vi "Read DisplayConfig.vi"(8 "error in":errorcluster caption="错误输入（无错误）", 11 "PCM PanelSplit 输入":refnum<class "PCM PanelSplit.lvclass"> caption="DNL_LabVIEW Object in") -> (0 "error out":errorcluster caption="错误输出", 2 "Display Config":T1={"Display Mode"=enum."时域", "ChTag[]"=[], "window"=1, "Range"={"Minimum"=0.0, "Maximum"=0.0, "Increment"=0.0, "Minor Increment"=0.0, "Start"=0.0}} {"window" items=["Rectangle"=0, "Hanning"=1, "Hamming"=2, "Blackman-Harris"=3, "Exact Blackman"=4, "Blackman"=5, "Flat Top"=6, "4 Term B-Harris "=7, "7 Term B-Harris"=8, "Low Sidelobe"=9, "Blackman Nuttall"=11, "Triangle"=30, "Bartlett-Hanning"=31, "Bohman"=32, "Parzen"=33, "Welch"=34, "Kaiser"=60, "Dolph-Chebyshev"=61, "Gaussian"=62]}, 3 "PCM PanelSplit 输出":refnum<class "PCM PanelSplit.lvclass"> caption="DNL_LabVIEW Object out")   [LabVIEW 2016, in "PCM PanelSplit.lvclass"]
uses:
  PCM PanelSplit.lvclass
  Display Config.ctl
  Display Mode.ctl
  <vilib>/Analysis/4window.llb/windowTd.ctl
  <vilib>/Utility/miscctls.llb/LVRangeTypeDef.ctl
  <vilib>/Analysis/NI_AALPro.lvlib
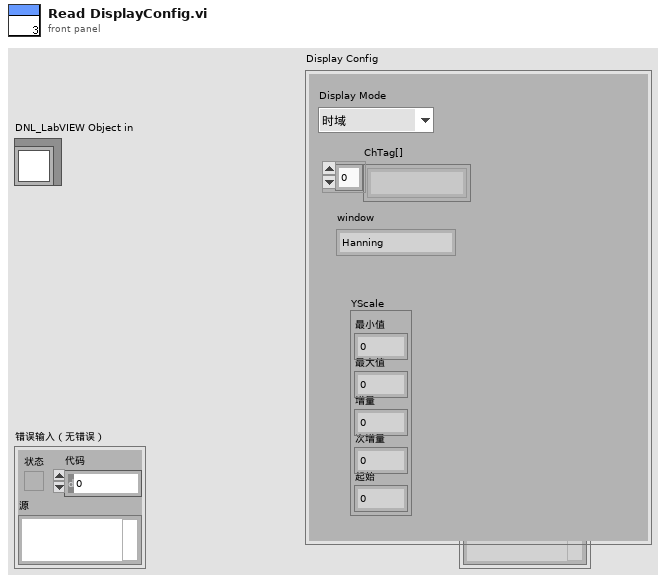
[diagram p1: front panel]
types:
  T1 = typedef "PCM PanelSplit.lvclass/Display Config.ctl" = cluster{"Display Mode":T2, "ChTag[]":string[], "window":T3, "Range":T4}
  T2 = typedef "PCM PanelSplit.lvclass/Display Mode.ctl" = enum16{"时域", "频谱", "功率谱"}
  T3 = typedef "NI_AALPro.lvlib/windowTd.ctl" = u32
  T4 = typedef "LVRangeTypeDef.ctl" = cluster{"Minimum":dbl, "Maximum":dbl, "Increment":dbl, "Minor Increment":dbl, "Start":dbl}
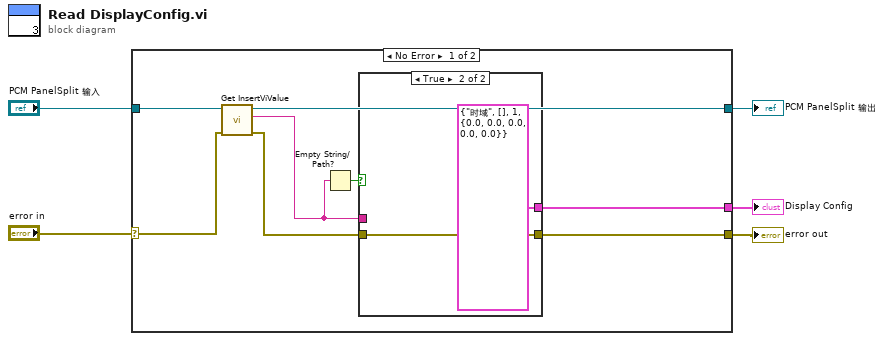
[diagram p0: block diagram]
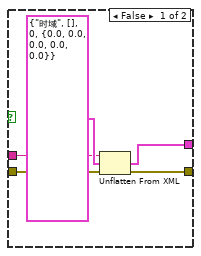
[diagram p2: hidden frame]
diagram:
  n1 = case shown="No Error" "error in" {
    selector: "error in" -> [w10 w22]
    tunnel: [w9 w22] -> w4
    tunnel: [w12 w21] -> w2
    tunnel: "PCM PanelSplit 输入" -> [w13 w21]
    tunnel: [w8 _] -> w1
    frame No Error {
      n2 = call-dynamic "Get InsertViValue.vi"("error in (no error)"=w10, "PanelDataNode 输入"=w13) -> ("error out"=w11:errorcluster, "ViValue"=w7:string, "PanelDataNode 输出"=w12:refnum<class "PCM PanelSplit.lvclass">)  [unwired: 7 in]
      n3 = Empty String/Path?(string/path=w7) -> (empty?=w6:bool)
      n4 = case shown="True" w6 {
        tunnel: w11 -> [w17 w20]
        tunnel: [w16 w20] -> w9
        tunnel: [w15 T1 {"Display Mode"=enum."时域", "ChTag[]"=[], "window"=1, "Range"={"Minimum"=0.0, "Maximum"=0.0, "Increment"=0.0, "Minor Increment"=0.0, "Start"=0.0}} ("Display Config")] -> w8
        tunnel: w7 -> [w14 _]
        frame False {
          n5 = Unflatten From XML(xml string=w14, type=T1 {"Display Mode"=enum."时域", "ChTag[]"=[], "window"=0, "Range"={"Minimum"=0.0, "Maximum"=0.0, "Increment"=0.0, "Minor Increment"=0.0, "Start"=0.0}} ("Display Config"), error in (no error)=w17) -> (value=w15:T1, error out=w16:errorcluster)
        }
        frame True {
        }
      }
    }
    frame Error {
    }
  }
  "error out" <- w4
  "PCM PanelSplit 输出" <- w2
  "Display Config" <- w1
